vi "ColorDetect1.0.vi"(8 "error in (no error)":errorcluster, 9 "Color Upper":T1, 10 "Color Lower":T1, 11 "new picture":picture) -> (0 "error out":errorcluster, 1 "found":u32[][](array[numeric]), 2 "image":u8[][](array[numeric]), 3 "out picture":picture)   [LabVIEW 2014, in "QwaveSys Raspberry Pi Library.lvlib"]
uses:
  QwaveSys Raspberry Pi Library.lvlib
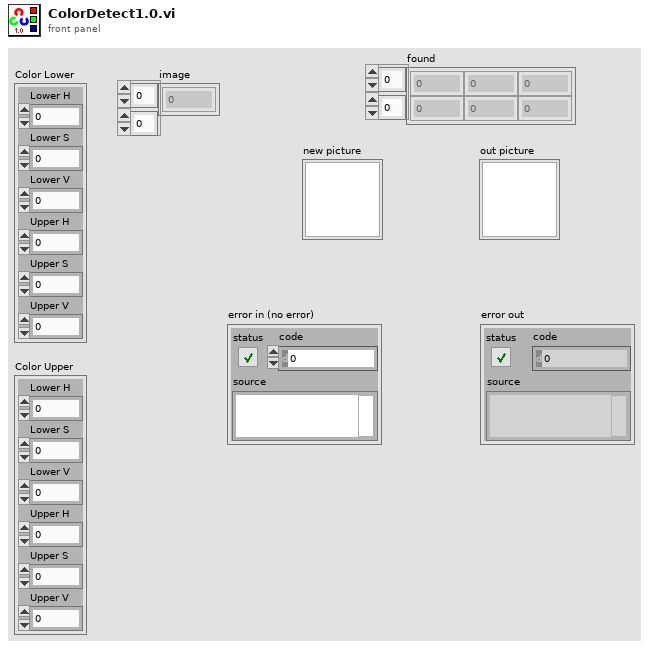
[diagram p1: front panel]
types:
  T1 = cluster{"Lower H":u8, "Lower S":u8, "Lower V":u8, "Upper H":u8, "Upper S":u8, "Upper V":u8}
  T2 = cluster{"Width":u16, "Style":enum32{"Solid", "Dash", "Dot", "DashDot", "DashDotDot"}}
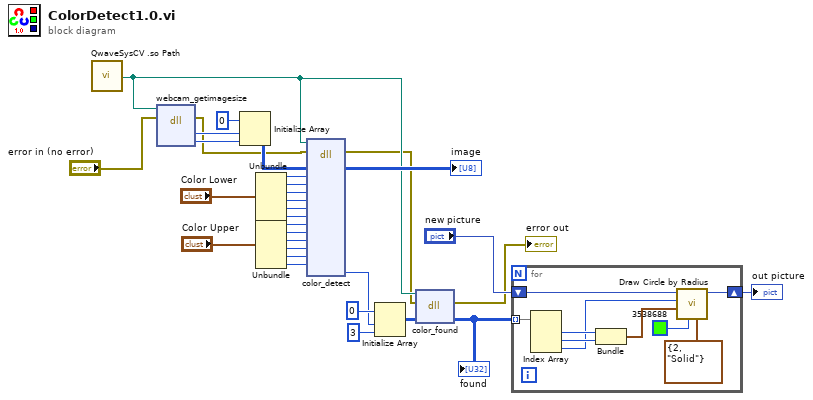
[diagram p0: block diagram]
diagram:
  n1 = call "QwaveSysCV .so Path.vi"() -> ("QwaveSys .so Path"=w4:path)  [unwired: 5 in]
  n2 = dll-call lib="libqwavesys.so" fn="webcam_getimagesize"(path in=w4, error in="error in (no error)") -> (error out=w5:errorcluster, "rows"=w30:i32, "cols"=w31:i32)  [unwired: 4 in, 1 out]
  n3 = Initialize Array(u8 0 ("element"), w30, w31) -> (w29:u8[][])
  n4 = Unbundle("Color Lower") -> ("Lower H"=w16:u8, "Lower S"=w17:u8, "Lower V"=w18:u8, "Upper H"=w19:u8, "Upper S"=w20:u8, "Upper V"=w21:u8)
  n5 = Unbundle("Color Upper") -> ("Lower H"=w23:u8, "Lower S"=w24:u8, "Lower V"=w25:u8, "Upper H"=w26:u8, "Upper S"=w27:u8, "Upper V"=w28:u8)
  n6 = dll-call lib="libqwavesys.so" fn="color_detect"(path in=w4, error in=w5, "image"=w29, "Alower_h"=w16, "Alower_s"=w17, "Alower_v"=w18, "Aupper_h"=w19, "Aupper_s"=w20, "Aupper_v"=w21, "Blower_h"=w23, "Blower_s"=w24, "Blower_v"=w25, "Bupper_h"=w26, "Bupper_s"=w27, "Bupper_v"=w28) -> (error out=w3:errorcluster, "image"=→"image":u8[][], "found"=w6:i32)  [unwired: 15 in, 1 out]
  n7 = Initialize Array(u32 0 ("element"), w6, 3 ("dimension size")) -> (w10:u32[][])
  n8 = dll-call lib="libqwavesys.so" fn="color_found"(path in=w4, error in=w3, "found"=w10) -> (error out=→"error out":errorcluster, "found"=w9:u32[][])  [unwired: 2 in, 1 out]
  "found" <- w9
  n9 = for {
    tunnel: w9 -> [w38] mode=indexing
    shift-right: [w32] -> w7
    shift-left: "new picture" -> [w33]
    n10 = Index Array(array=w38) -> (element #1=w37:u32, element #2=w36:u32, element #3=w35:u32)  [unwired: 3 in]
    n11 = Bundle(w37, w36) -> (w40:cluster{u32, u32})  [unwired: 1 in]
    n12 = call <vilib>:"Draw Circle by Radius.vi"("pen"=T2 {"Width"=2, "Style"=enum."Solid"}, "color(black)"=u32 3538688, "pixel center"=w40, "radius"=w35, "picture"=w33) -> ("new picture"=w32:picture)  [unwired: 6 in]
  }
  "out picture" <- w7
